vi "Main.vi"() -> ()   [LabVIEW 2011]
panel:
  in  "stop":bool
  in  "OK_Visualiza":bool
  in  "OK_Analiza":bool
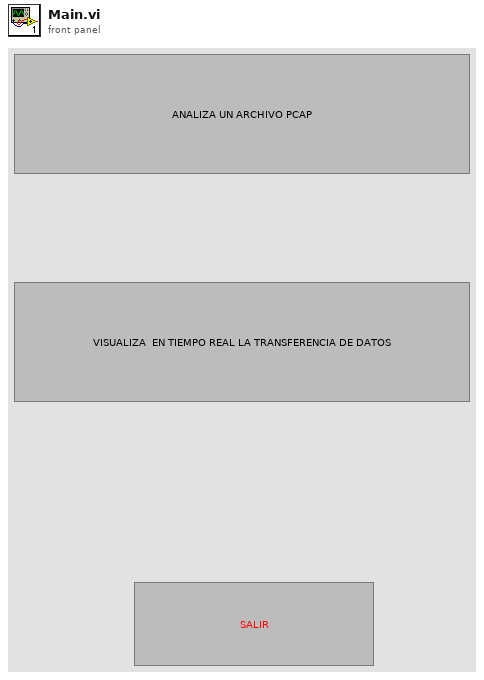
[diagram p1: front panel]
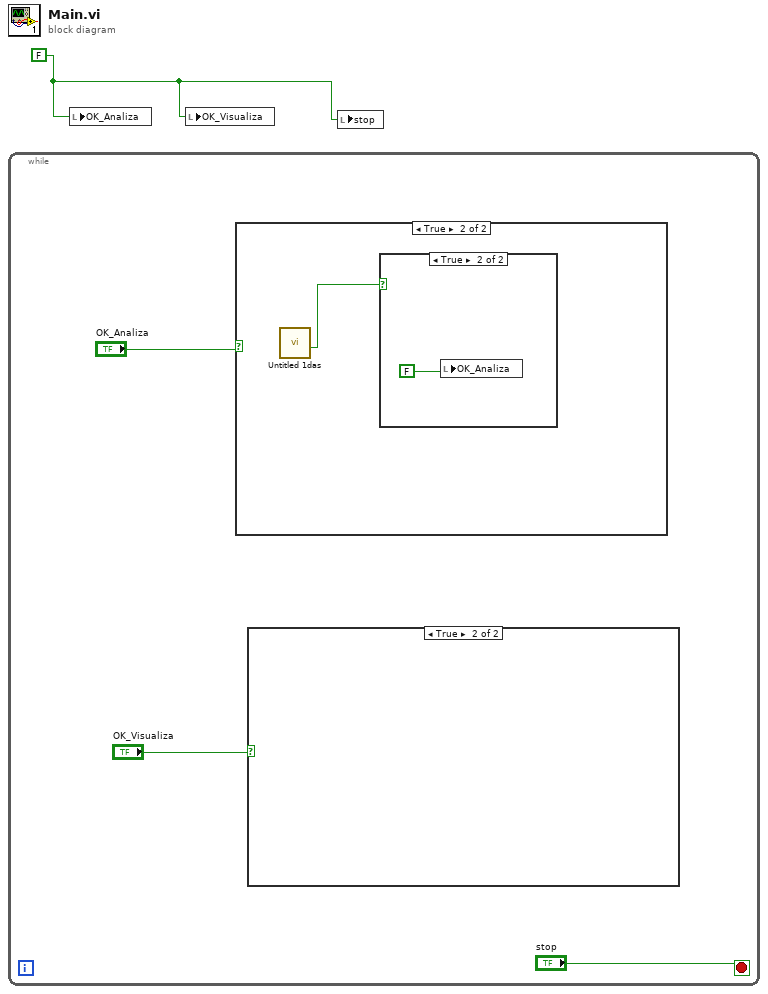
[diagram p0: block diagram]
diagram:
  w1 = FALSE
  n1 = while {
    stop <- "stop" stop-if-true
    n2 = case shown="True" "OK_Analiza" {
      frame False {
      }
      frame True {
        n3 = call "Untitled 1das.vi"() -> ("Salir 2"=w5:bool)  [unwired: 11 in]
        n4 = case shown="True" w5 {
          frame False {
          }
          frame True {
            n5 = local write "OK_Analiza"(FALSE) -> ()
          }
        }
      }
    }
    n6 = case shown="True" "OK_Visualiza" {
      frame False {
      }
      frame True {
      }
    }
  }
  n7 = local write "OK_Analiza"(w1) -> ()
  n8 = local write "OK_Visualiza"(w1) -> ()
  n9 = local write "stop"(w1) -> ()
